vi "Intake main.vi"() -> ()   [LabVIEW 2018]
uses:
  <vilib>/Rock Robotics/WPI/ThirdParty/Phoenix-LabVIEW/Motor Controller/Controls/CTRE_Phoenix_MotorControl_ControlMode.ctl
  <vilib>/Rock Robotics/WPI/Solenoid/Deprecated/WPI_SolenoidSetBool.vi
  Robot Global Data.vi
panel:
  out "Hatch Right":bool
  out "Hatch Left":bool
  out "Ball Inside?":bool
  in  "Push":bool
  in  "Clamp":bool
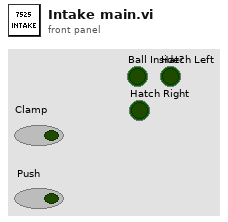
[diagram p1: front panel]
types:
  T1 = typedef "CTRE_Phoenix_MotorControl_ControlMode.ctl" = u16
  T2 = typedef "WPI_DigitalInputDevRef.ctl" = cluster{"DevStatus":errorcluster, "DIO Channel":T3}
  T3 = typedef "FPGA_DIOChannel.ctl" = enum8{"DIO 0", "DIO 1", "DIO 2", "DIO 3", "DIO 4", "DIO 5", "DIO 6", "DIO 7", "DIO 8", "DIO 9", "DIO MXP 0", "DIO MXP 1", "DIO MXP 2", "DIO MXP 3", "DIO MXP 4", "DIO MXP 5", "DIO MXP 6", "DIO MXP 7", "DIO MXP 8", "DIO MXP 9", "DIO MXP 10", "DIO MXP 11", "DIO MXP 12", "DIO MXP 13", "DIO MXP 14", "DIO MXP 15", "SPI Port CS1", "SPI Port CS2", "SPI Port CS3", "SPI Port MISO", "SPI Port MOSI", "Invalid"}
  T4 = typedef "WPI_SolenoidDevRef.ctl" = cluster{"DevStatus":errorcluster, "Pneumatics Control Module":u8, "Forward Solenoid Channel":T5, "Reverse Solenoid Channel":T5}
  T5 = typedef "WPI_SolenoidChannel.ctl" = enum8{"Solenoid 0", "Solenoid 1", "Solenoid 2", "Solenoid 3", "Solenoid 4", "Solenoid 5", "Solenoid 6", "Solenoid 7", "Invalid"}
  T6 = typedef "WPI_MotorControlDeviceRef.ctl" = cluster{"DeviceStatus":errorcluster, "Type":T7, "PWM":cluster{"PWM Channel":T8, "DeadBand":T9}, "CAN":cluster{"Device Number":u8, "SetOutput VI Ref":variant, "GetOutput VI Ref":variant, "Enable VI Ref":variant, "Disable VI Ref":variant, "Data":variant}, "Invert":bool, "DIO PWM":cluster{"PWM \"Enable\" Channel":T8, "DIOChannel":T3, "PWM Rate":dbl}}
  T7 = typedef "WPI_MotorControlType.ctl" = enum16{"PWM", "CAN", "DIO PWM"}
  T8 = typedef "FPGA_DIOPWMChannel.ctl" = enum8{"PWM 0", "PWM 1", "PWM 2", "PWM 3", "PWM 4", "PWM 5", "PWM 6", "PWM 7", "PWM 8", "PWM 9", "PWM MXP 0", "PWM MXP 1", "PWM MXP 2", "PWM MXP 3", "PWM MXP 4", "PWM MXP 5", "PWM MXP 6", "PWM MXP 7", "PWM MXP 8", "PWM MXP 9", "Invalid"}
  T9 = typedef "WPI_PWMDeadband.ctl" = cluster{"Name":string, "maxPositivePwm":i32, "minPositivePwm":i32, "centerPwm":i32, "maxNegativePwm":i32, "minNegativePwm":i32, "angularRange":u16}
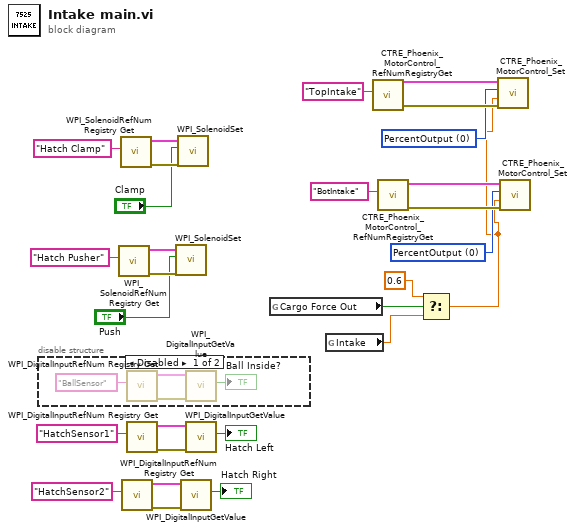
[diagram p0: block diagram]
diagram:
  w13 = T1 0 items=["PercentOutput"=0, "Position"=1, "Velocity"=2, "Current"=3, "Follower"=5, "MotionProfile"=6, "MotionMagic"=7, "MotionProfileArc"=10, "Disabled"=15] ("Control Mode")
  w14 = T1 0 items=["PercentOutput"=0, "Position"=1, "Velocity"=2, "Current"=3, "Follower"=5, "MotionProfile"=6, "MotionMagic"=7, "MotionProfileArc"=10, "Disabled"=15] ("Control Mode")
  n1 = disable-structure shown="Disabled" {
    frame Disabled {
      n2 = call <vilib>:"WPI_DigitalInputRefNum Registry Get.vi"("refnum name"="BallSensor") -> ("error out"=w32:errorcluster, "DigitalInputDevRef"=w31:T2)  [unwired: 9 in]
      n3 = call <vilib>:"WPI_DigitalInputGetValue.vi"("error in (no error)"=w32, "DigitalInputDevRef"=w31) -> ("Value"=→"Ball Inside?":bool)  [unwired: 7 in, 2 out]
    }
    frame Enabled {
    }
  }
  n4 = call <vilib>:"WPI_SolenoidRefNum Registry Get.vi"("refnum name"="Hatch Pusher") -> ("error out"=w23:errorcluster, "SolenoidDevRef"=w24:T4)  [unwired: 9 in]
  n5 = call <vilib>:"WPI_SolenoidRefNum Registry Get.vi"("refnum name"="Hatch Clamp") -> ("error out"=w28:errorcluster, "SolenoidDevRef"=w27:T4)  [unwired: 9 in]
  n6 = call <vilib>:"WPI_DigitalInputRefNum Registry Get.vi"("refnum name"="HatchSensor2") -> ("error out"=w9:errorcluster, "DigitalInputDevRef"=w8:T2)  [unwired: 9 in]
  n7 = call <vilib>:"WPI_DigitalInputRefNum Registry Get.vi"("refnum name"="HatchSensor1") -> ("error out"=w10:errorcluster, "DigitalInputDevRef"=w11:T2)  [unwired: 9 in]
  n8 = call-poly <vilib>:"WPI_SolenoidSet.vi"("error in (no error)"=w23, "Value"="Push", "SolenoidDevRef"=w24) -> ()  [unwired: 7 in, 2 out]
  n9 = call-poly <vilib>:"WPI_SolenoidSet.vi"("error in (no error)"=w28, "Value"="Clamp", "SolenoidDevRef"=w27) -> ()  [unwired: 7 in, 2 out]
  n10 = call <vilib>:"WPI_DigitalInputGetValue.vi"("error in (no error)"=w9, "DigitalInputDevRef"=w8) -> ("Value"=→"Hatch Right":bool)  [unwired: 7 in, 2 out]
  n11 = call <vilib>:"WPI_DigitalInputGetValue.vi"("error in (no error)"=w10, "DigitalInputDevRef"=w11) -> ("Value"=→"Hatch Left":bool)  [unwired: 7 in, 2 out]
  n12 = global read "Robot Global Data.vi" "Cargo Force Out"() -> (w4:bool)
  n13 = global read "Robot Global Data.vi" "Intake"() -> (w1:dbl)
  n14 = call <vilib>:"CTRE_Phoenix_MotorControl_RefNumRegistryGet.vi"("refnum name"="TopIntake") -> ("error out"=w17:errorcluster, "PhoenixMotorControlDevRef"=w18:T6)  [unwired: 9 in]
  n15 = call <vilib>:"CTRE_Phoenix_MotorControl_RefNumRegistryGet.vi"("refnum name"="BotIntake") -> ("error out"=w15:errorcluster, "PhoenixMotorControlDevRef"=w16:T6)  [unwired: 9 in]
  n16 = Select(t=0.6, s=w4, f=w1) -> (s? t:f=w2:dbl)
  n17 = call <vilib>:"CTRE_Phoenix_MotorControl_Set.vi"("error in (no error)"=w17, "Output"=w2, "Control Mode"=w14, "PhoenixMotorControlDevRef"=w18) -> ()  [unwired: 6 in, 2 out]
  n18 = call <vilib>:"CTRE_Phoenix_MotorControl_Set.vi"("error in (no error)"=w15, "Output"=w2, "Control Mode"=w13, "PhoenixMotorControlDevRef"=w16) -> ()  [unwired: 6 in, 2 out]
